vi "CRYText entry dialog multi-line.vi"(0 "text":string, 1 "Text":string, 4 "Title Name":string) -> (7 "text entered":string, 10 "Cancelled?":bool)   [LabVIEW 2013]
panel:
  in  "OK":bool
  in  "Cancel":bool
  out "Dialog Text":string
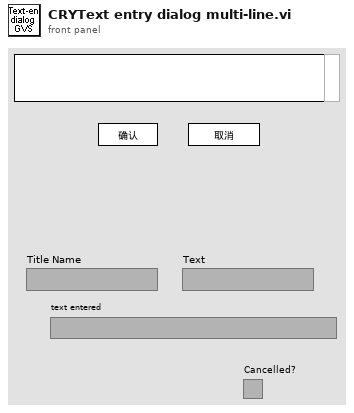
[diagram p1: front panel]
types:
  T1 = enum16{"OK", "Yes", "YesNo", "YesNoCancel", "ReplaceAppend"}
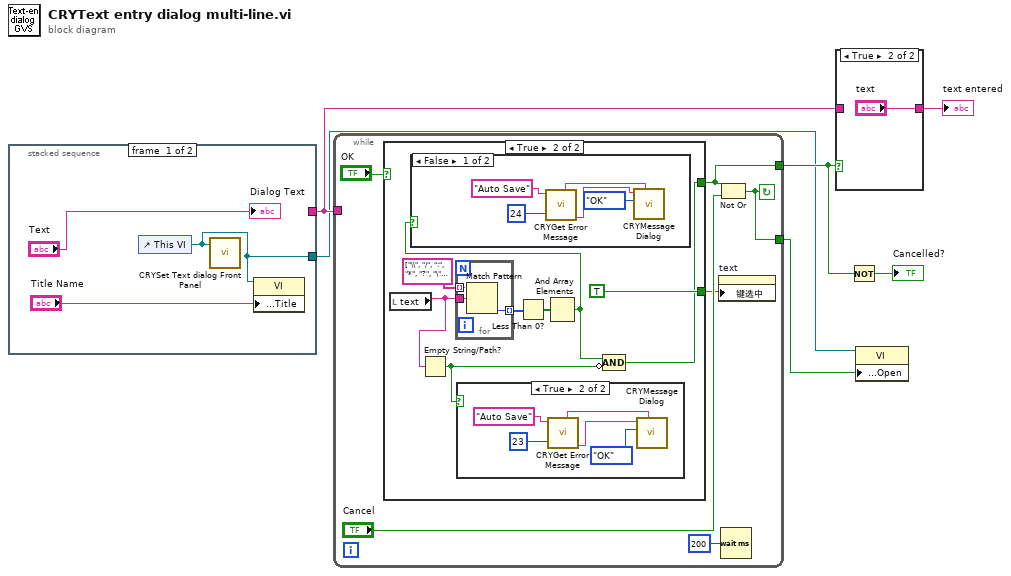
[diagram p0: block diagram]
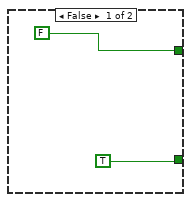
[diagram p2: hidden frame]
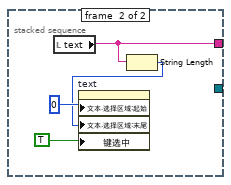
[diagram p5: hidden frame]
diagram:
  n1 = stacked-sequence {
    tunnel: [_ w13] -> w5
    tunnel: [w9 _] -> w2
    frame #0 {
      n2 = control-ref of="This VI"() -> (w9:refnum<vi>)
      n3 = call "CRYSet Text dialog Front Panel.vi"("Vi Ref"=w9) -> ()  [unwired: 11 in]
      n4 = property class="VI"(reference=w9, "Front Panel.Title"="Title Name") -> ()  [unwired: 1 in, 2 out]
      "Dialog Text" <- "Text"
    }
    frame #1 {
      n5 = local read "text"() -> (w13:string)
      n6 = String Length(string=w13) -> (length=w11:i32)
      n7 = property on="text" class="Str"("文本.选择区域:起始"=u32 0 ("Selection Start"), "文本.选择区域:末尾"=w11, "键选中"=TRUE ("Key Focus")) -> ()  [unwired: 2 in, 2 out]
    }
  }
  n8 = while {
    tunnel: w5 -> [_]
    tunnel: [w16] -> w4
    tunnel: [w14] -> w1
    stop <- w14 continue-if-true
    n9 = case shown="True" "OK" {
      tunnel: [FALSE w22] -> w16
      tunnel: [TRUE TRUE ("Key Focus")] -> w15
      frame False {
      }
      frame True {
        n10 = local read "text"() -> (w26:string)
        n11 = Empty String/Path?(string/path=w26) -> (empty?=w24:bool)
        n12 = for {
          tunnel: w26 -> [w42]
          tunnel: string[] ["\\", "/", ":", "*", "?", "\"", "<", ">", "|"] ("1D array") -> [w41] mode=indexing
          tunnel: [w40] -> w28 mode=indexing
          n13 = Match Pattern(string=w42, regular expression=w41) -> (offset past match=w40:i32)  [unwired: 1 in, 3 out]
        }
        n14 = case shown="True" w24 {
          frame False {
          }
          frame True {
            n15 = call "CRYGet Error Message.vi"("Error No"=23, "Kind"="Auto Save") -> ("Message Sub 3"=w32:string, "Window Title"=w31:string)  [unwired: 4 in, 4 out]
            n16 = call "CRYMessage Dialog.vi"("Window Title"=w31, "YesNoCancel"=T1."OK", "Message Content"=w32) -> ()  [unwired: 7 in, 2 out]
          }
        }
        n17 = Less Than 0?(x=w28) -> (x < 0?=w27:bool[])
        n18 = And Array Elements(Boolean array=w27) -> (logical AND=w23:bool)
        n19 = case shown="False" w23 {
          frame False {
            n20 = call "CRYGet Error Message.vi"("Error No"=24, "Kind"="Auto Save") -> ("Message Sub 3"=w36:string, "Window Title"=w37:string)  [unwired: 4 in, 4 out]
            n21 = call "CRYMessage Dialog.vi"("Window Title"=w37, "YesNoCancel"=T1."OK", "Message Content"=w36) -> ()  [unwired: 7 in, 2 out]
          }
          frame True {
          }
        }
        n22 = Compound Arithmetic op=AND(w23, invert w24) -> (w22:bool)
      }
    }
    n23 = Not Or(1:"Cancel", 2:w16) -> (0:w14:bool)
    n24 = property on="text" class="Str"("键选中"=w15) -> ()  [unwired: 2 in, 2 out]
    n25 = Wait (ms)(milliseconds to wait=u32 200) -> ()  [unwired: 1 out]
  }
  n26 = case shown="True" w4 {
    tunnel: [w43 "text"] -> w6
    tunnel: w5 -> [w43 _]
    frame False {
    }
    frame True {
    }
  }
  "text entered" <- w6
  n27 = Not(x=w4) -> (.not. x?=→"Cancelled?":bool)
  n28 = property class="VI"(reference=w2, "Front Panel.Open"=w1) -> ()  [unwired: 1 in, 2 out]
